vi "Delay & unit to delay (s).vi"(1 "OverallPeriod":dbl[unit], 2 "Delay Value":dbl, 3 "Delay Unit":u16) -> (0 "Delay (s)":dbl[unit])   [LabVIEW 2017, in "Pulse Generator.lvclass"]
uses:
  Pulse Generator.lvclass
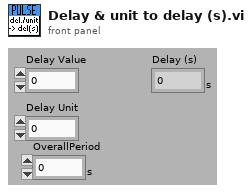
[diagram p1: front panel]
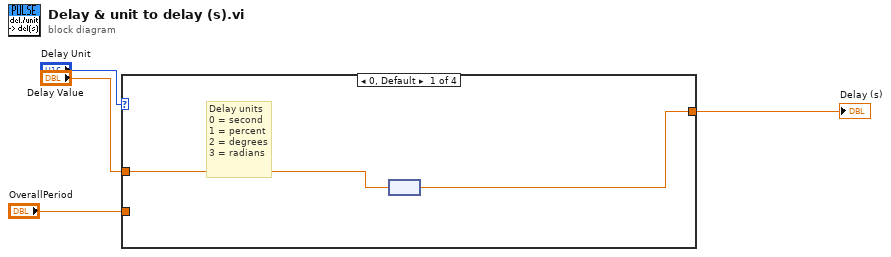
[diagram p0: block diagram]
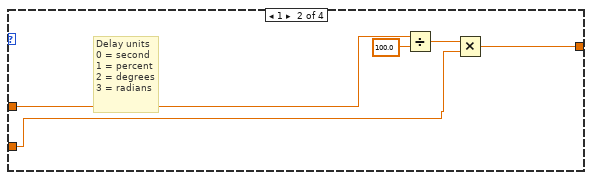
[diagram p2: hidden frame]
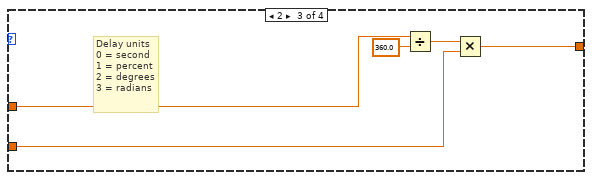
[diagram p3: hidden frame]
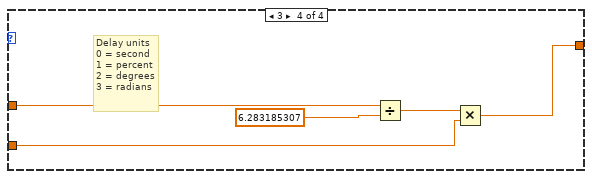
[diagram p4: hidden frame]
diagram:
  n1 = case shown="0, Default" "Delay Unit" {
    tunnel: "Delay Value" -> [w6 w10 w14 w19]
    tunnel: [w5 w8 w13 w18] -> w3
    tunnel: "OverallPeriod" -> [_ w7 w12 w17]
    frame 0, Default {
      # "Delay units\n0 = second\n1 = percent\n2 = degrees\n3 = radians"
      n2 = node(w6) -> (w5:dbl[unit])
    }
    frame 1 {
      # "Delay units\n0 = second\n1 = percent\n2 = degrees\n3 = radians"
      n3 = Divide(x=w10, y=100.0) -> (x/y=w9:dbl)
      n4 = Multiply(x=w9, y=w7) -> (x*y=w8:dbl[unit])
    }
    frame 2 {
      # "Delay units\n0 = second\n1 = percent\n2 = degrees\n3 = radians"
      n5 = Divide(x=w14, y=360.0) -> (x/y=w15:dbl)
      n6 = Multiply(x=w15, y=w12) -> (x*y=w13:dbl[unit])
    }
    frame 3 {
      # "Delay units\n0 = second\n1 = percent\n2 = degrees\n3 = radians"
      n7 = Divide(x=w19, y=6.283185307) -> (x/y=w20:dbl)
      n8 = Multiply(x=w20, y=w17) -> (x*y=w18:dbl[unit])
    }
  }
  "Delay (s)" <- w3
